vi "Global PLC Ref.vi"(8 "error in (no error)":errorcluster, 9 "Operation Siemens Ref":T3=enum."Add Ref", 10 "IP Address":string, 11 "Siemens Ctr":T1) -> (0 "error out":errorcluster, 1 "semaphore":T2, 2 "Boolean":bool, 3 "Siemens Ctr out":T1, 4 "PLC Ref":T1[](array[typedef]))   [LabVIEW 2014, in "Simatic S7.lvlib"]
uses:
  Simatic S7.lvlib
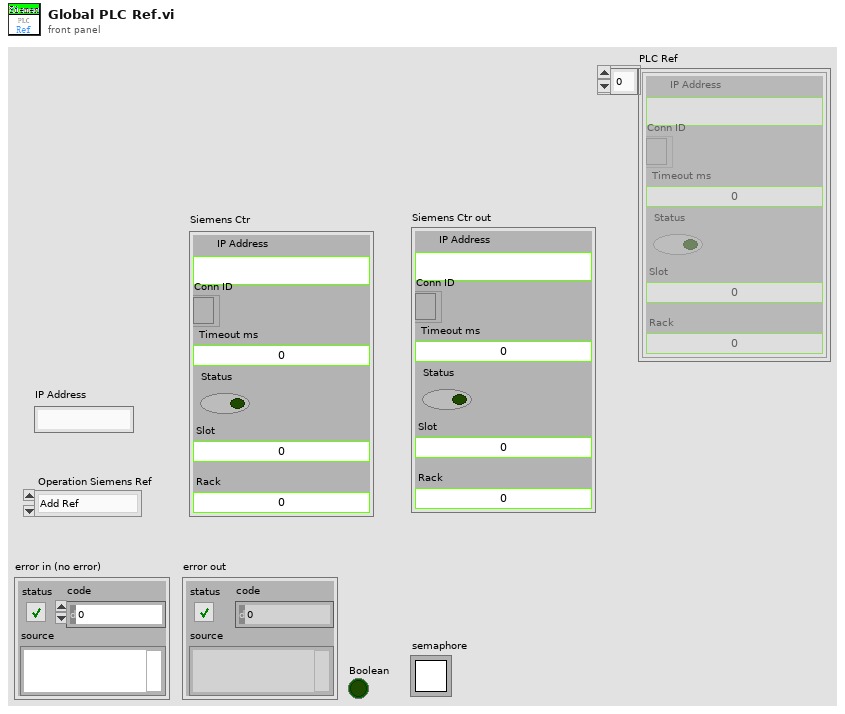
[diagram p1: front panel]
types:
  T1 = typedef "Simatic S7.lvlib/Siemens Ref.ctl" = cluster{"IP Address ":string, "Conn ID":refnum<k5>, "Timeout ms":i32, "Status":bool, "Slot":u16, "Rack":u16}
  T2 = typedef "Semaphore RefNum" = refnum<k1>
  T3 = typedef "Simatic S7.lvlib/Operation Siemens Ref.ctl" = enum16{"Init", "Add Ref", "Get Ref", "Set Error", "Close Close"}
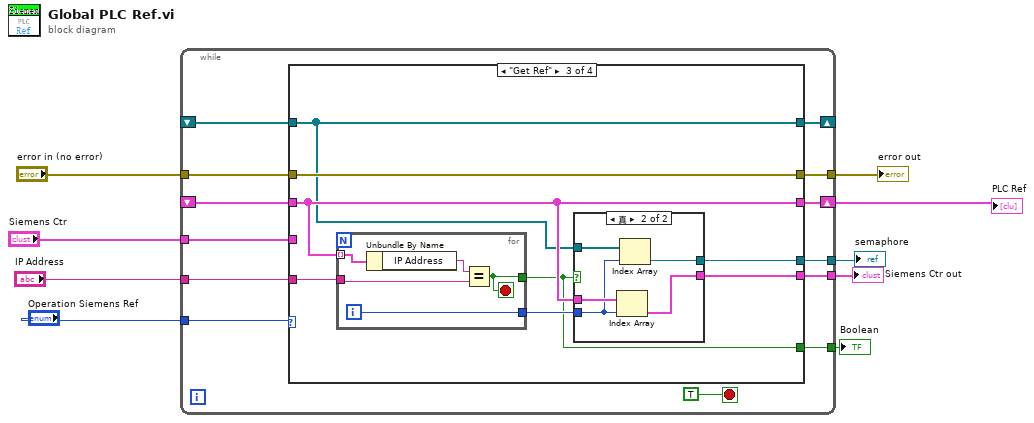
[diagram p0: block diagram]
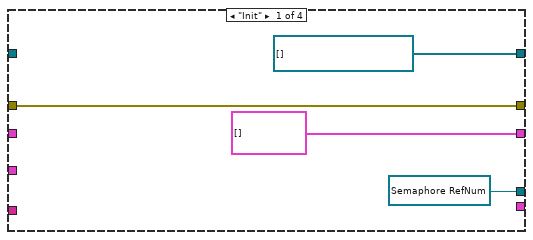
[diagram p2: hidden frame]
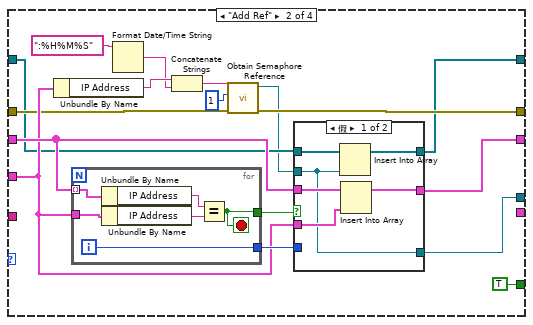
[diagram p3: hidden frame]
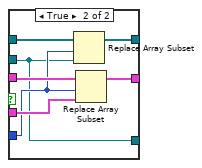
[diagram p4: hidden frame]
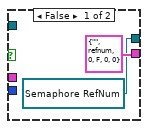
[diagram p5: hidden frame]
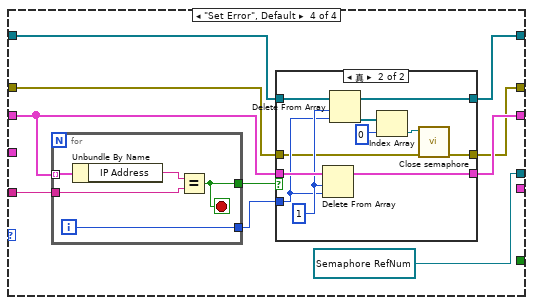
[diagram p6: hidden frame]
diagram:
  n1 = while {
    tunnel: "Siemens Ctr" -> [w18]
    tunnel: "IP Address" -> [w21]
    shift-right: [w20] -> w1
    shift-left: _ -> [w19]
    tunnel: [w17] -> w7
    tunnel: [w16] -> w6
    shift-right: [w15] -> _
    shift-left: _ -> [w14]
    tunnel: "error in (no error)" -> [w13]
    tunnel: [w12] -> w4
    tunnel: [w11] -> w3
    tunnel: "Operation Siemens Ref" -> [w10]
    stop <- TRUE stop-if-true
    n2 = case shown="\"Get Ref\"" w10 {
      tunnel: w21 -> [_ _ w70 w92]
      tunnel: [T1[] [] ("PLC Ref") w40 w69 w88] -> w20
      tunnel: w19 -> [_ w41 w69 w89]
      tunnel: w18 -> [_ w39 _ _]
      tunnel: [_ _ w67 _] -> w17
      tunnel: [_ TRUE w66 _] -> w16
      tunnel: [w24 w33 w64 w86] -> w15
      tunnel: w14 -> [_ w36 w64 w87]
      tunnel: w13 -> [w25 w38 w65 w85]
      tunnel: [w25 w37 w65 w84] -> w12
      tunnel: [w23 w29 w63 w83] -> w11
      frame "Init" {
        w23 = T2 refnum items=["semaphore"] ("semaphore")
        w24 = T2[] [] items=["semaphore"]
      }
      frame "Add Ref" {
        n3 = Unbundle By Name(w39) -> ("IP Address"=w31:string)
        n4 = for {
          tunnel: w41 -> [w62] mode=indexing
          tunnel: w39 -> [w58]
          tunnel: [w60] -> w42
          tunnel: [w59] -> w43
          i -> [w60]
          stop <- w59 stop-if-true
          n5 = Unbundle By Name(w62) -> ("IP Address"=w61:string)
          n6 = Unbundle By Name(w58) -> ("IP Address"=w57:string)
          n7 = Equal?(x=w61, y=w57) -> (x = y?=w59:bool)
        }
        n8 = Format Date/Time String(time format string (%c)=":%H%M%S") -> (date/time string=w30:string)  [unwired: 2 in]
        n9 = Concatenate Strings(w31, w30) -> (w34:string)
        n10 = call <vilib>:"Obtain Semaphore Reference.vi"("error in (no error)"=w38, "size (1)"=1, "name (unnamed)"=w34) -> ("error out"=w37:errorcluster, "semaphore"=w32:T2)  [unwired: 2 in, 1 out]
        n11 = case shown="假" w43 {
          tunnel: w42 -> [_ w51]
          tunnel: w41 -> [w49 w56]
          tunnel: w39 -> [w47 w55]
          tunnel: [w48 w54] -> w40
          tunnel: w36 -> [w46 w53]
          tunnel: w32 -> [w44 w50]
          tunnel: [w45 w52] -> w33
          tunnel: [w44 w50] -> w29
          frame False {
            n12 = Insert Into Array(array=w46, new element=w44) -> (w45:T2[])  [unwired: 1 in]
            n13 = Insert Into Array(array=w49, new element=w47) -> (w48:T1[])  [unwired: 1 in]
          }
          frame True {
            n14 = Replace Array Subset(array=w53, new element=w50, index=w51) -> (w52:T2[])
            n15 = Replace Array Subset(array=w56, new element=w55, index=w51) -> (w54:T1[])
          }
        }
      }
      frame "Get Ref" {
        n16 = for {
          tunnel: w69 -> [w82] mode=indexing
          tunnel: w70 -> [w80]
          tunnel: [w79] -> w68
          tunnel: [w78] -> w66
          i -> [w79]
          stop <- w78 stop-if-true
          n17 = Unbundle By Name(w82) -> ("IP Address"=w81:string)
          n18 = Equal?(x=w81, y=w80) -> (x = y?=w78:bool)
        }
        n19 = case shown="真" w66 {
          tunnel: w69 -> [_ w77]
          tunnel: w68 -> [_ w74]
          tunnel: [T1 {"IP Address "="", "Conn ID"=refnum, "Timeout ms"=0, "Status"=FALSE, "Slot"=0, "Rack"=0} ("Siemens Ctr") w76] -> w67
          tunnel: w64 -> [_ w75]
          tunnel: [w71 w73] -> w63
          frame False {
            w71 = T2 refnum items=["semaphore"] ("semaphore")
          }
          frame True {
            n20 = Index Array(array=w77, index=w74) -> (element=w76:T1)
            n21 = Index Array(array=w75, index=w74) -> (element=w73:T2)
          }
        }
      }
      frame "Set Error", Default {
        w83 = T2 refnum items=["semaphore"] ("semaphore")
        n22 = for {
          tunnel: w89 -> [w111] mode=indexing
          tunnel: w92 -> [w109]
          tunnel: [w108] -> w91
          tunnel: [w107] -> w90
          i -> [w107]
          stop <- w108 stop-if-true
          n23 = Unbundle By Name(w111) -> ("IP Address"=w110:string)
          n24 = Equal?(x=w110, y=w109) -> (x = y?=w108:bool)
        }
        n25 = case shown="真" w91 {
          tunnel: w90 -> [_ w102]
          tunnel: w89 -> [w95 w106]
          tunnel: [w95 w105] -> w88
          tunnel: w87 -> [w94 w104]
          tunnel: [w94 w101] -> w86
          tunnel: w85 -> [w93 w98]
          tunnel: [w93 w96] -> w84
          frame False {
          }
          frame True {
            w103 = 1 ("length")
            n26 = Delete From Array(array=w106, length=w103, index=w102) -> (array with subset deleted=w105:T1[])  [unwired: 1 out]
            n27 = Delete From Array(array=w104, length=w103, index=w102) -> (deleted portion=w100:T2[], array with subset deleted=w101:T2[])
            n28 = Index Array(array=w100, index=0) -> (element=w97:T2)
            n29 = call "Close semaphore.vi"("error in (no error)"=w98, "semaphore"=w97) -> ("error out"=w96:errorcluster)  [unwired: 8 in, 1 out]
          }
        }
      }
    }
  }
  "Boolean" <- w6
  "Siemens Ctr out" <- w7
  "error out" <- w4
  "semaphore" <- w3
  "PLC Ref" <- w1
